vi "cs-scanning_v5_ssx.vi"() -> ()   [LabVIEW 2017]
uses:
  fpga_subVIs_ssxy/fixed-point-ss/typeDefs/FXPControlParams-ss-xy.ctl
  controls/supervisor-params.ctl
  controls/fpga-scan-status.ctl
  controls/boolean_info.ctl
  controls/z-axis-params_v4_prescan.ctl
  controls/TF-params.ctl
  <vilib>/Platform/TimedLoop/XDataNode/timing_clust.ctl
  <vilib>/Platform/TimedLoop/XDataNode/nitl_modes.ctl
  <vilib>/Platform/TimedLoop/XDataNode/wakeup.ctl
  <vilib>/rvi/Emulation/niFpgaGetClockAttributes.vi
  <vilib>/rvi/Emulation/niFpgaSctlEmulationGetInTimedLoop.vi
  <vilib>/rvi/Emulation/niFpgaEmulationReportErrorSimple.vi
  <vilib>/rvi/eio/common/nirviEmuTemplateMethod_errors.vi
  <vilib>/rvi/Emulation/niFpgaCriticalErrorInLSC.vi
  <vilib>/rvi/Memory/Memory_Emulation/nirvimemoryFastEmulation.vi
  <vilib>/rvi/Memory/Memory_Emulation/nirvimemoryEmulation.vi
  <vilib>/rvi/Emulation/niFpgaEmulationIsFPGAContextNoSignature.vi
  <vilib>/rvi/DataTransferAndStorage/Container/Common/niFpgaContainerGetUniqueNameForEmu.vi
  <vilib>/rvi/Emulation/niFpgaProcessEmulError.vi
  <vilib>/rvi/errors/nirviReportUnexpectedCaseInternalError (U32).vi
  <vilib>/rvi/Memory/Memory_Emulation/niFpgaMemoryEmulationCacheClearOnFirstRun.vi
  <vilib>/rvi/Memory/Memory_Emulation/nirvimemoryEmulationManagerCache_MakeExclusive.vi
  <vilib>/rvi/Memory/Memory_Emulation/niFpgaMemoryEmulationValidateCache.vi
  <vilib>/rvi/Memory/Memory_Emulation/nirvimemoryEmulationManagerCache_InsertValue.vi
  <vilib>/Utility/error.llb/Clear Errors.vi
  <vilib>/rvi/Memory/Memory_Emulation/nirvimemoryEmulationManagerCache_ReleaseExclusive.vi
  <vilib>/rvi/Memory/Memory_Emulation/nirvimemoryEmulationManagerCache_GetValue.vi
  <vilib>/rvi/Memory/Memory_Emulation/nirvimemoryEmulationManagerCache_SetValue.vi
  <vilib>/rvi/DataTransferAndStorage/Container/Common/niFpgaContainerExecOnDevCompGetState.vi
  <vilib>/rvi/errors/niFpgaSetErrorForExecOnDevCompSimple.vi
  <vilib>/rvi/eio/common/nirviEmuReportErrorAndStop.vi
  <vilib>/rvi/FIFO/Fifo_Resource/nirvififoEmulationSetSize.vi
  <vilib>/rvi/FIFO/Fifo_Resource/nirviFifoEmulationQueueMgr.vi
  <instcachedir>/0/nirviFifoEmulationQueueMgr_E5CAEC123FF24DC58D834DCA3CDAA9B5.lvgen/nirviFifoEmulationQueueMgr_E5CAEC123FF24DC58D834DCA3CDAA9B5_001.vi
  <vilib>/rvi/FIFO/Fifo_Resource/nirvififoEmulationDetermineInputValidOut.vi
  <vilib>/rvi/FIFO/Fifo_Resource/nirvififoEmulationCreateLock.vi
  <vilib>/rvi/FIFO/Fifo_Resource/nirvififoEmulationObtainLock.vi
  <vilib>/rvi/FIFO/Fifo_Resource/nirvififoEmulationReleaseLock.vi
  <vilib>/rvi/occurrence/nirviWaitOnOccurrenceBase.vi
  <vilib>/rvi/errors/nirviReportUnexpectedCaseInternalError.vi
  <vilib>/rvi/interface/RandomDataEmulation/niFpgaRandomDataHandleErrors.vi
  <vilib>/eio/EIONode/EIONode.xnode
  <vilib>/Platform/TimedLoop/XDataNode/XDataNode.xnode
  <vilib>/rvi/DataTransferAndStorage/Container/XNode/niFpgaContainer.xnode
  <vilib>/rvi/DataTransferAndStorage/Register/Emulation/niFpgaRegisterEmulation.vi
  <vilib>/rvi/FIFO/Fifo_Resource/niFpgaFifoEmulationRefIn.vi
  FPGA-data-logging.lvlib
  libimaging-cs.lvlib
  <vilib>/Platform/TimedLoop/XDataNode/XDNodeRunTimeDep.lvlib
panel:
  in  "collect-0":bool
  out "setup-finished":bool
  out "state0-count":u64
  in  "stop":bool
  out "u_z saturated":bool
  in  "z_axis_params":T1={"z_u_max"=5.0, "setpoint_scan"=0.0, "Ki_scan"=0.001, "uz_safe"=0.0, "Kiz_down"=0.001, "setpoint_up"=0.0, "do_Dz"=FALSE, "PID_while_xy_move"=FALSE, "TF_params"={"TF_order"=0, "Num"=[0.0, 0.0, 0.0, 0.0, 0.0, 0.0, 0.0, 0.0, 0.0], "Den"=[0.0, 0.0, 0.0, 0.0, 0.0, 0.0, 0.0, 0.0, 0.0]}} {"Kiz_down" format="%#_13g"; "z_u_max" format="%#_13g"}
  out "scan-status":T3
  in  "state-machine-params":T5={"xy_settled_samples_threshold"=15, "xy_error_threshold"=0.01, "zup_err_threshold"=0.10000228881835938, "prescan_samples"=5000, "TOL"=0.3, "collect_all"=TRUE, "numEntities"=0} {"TOL" format="%#_13g"}
  in  "num-log-channels":i32
  out "SS FIFO TimeOut?":bool
  in  "ControlParams-ss-xy":T6={"umax"=3.0, "Ns_obs/cntrl"=0, "ref_f_VEC"=[0.0, 0.0], "du_max"=0.0, "Nbar"=0.0, "Nhyst"=0, "Nsat"=0, "Ndrift+1"=0, "Ki-y"=0.01}
  out "loop-stopped":bool
  out "xyZ_k":fxp<+/-,16,5>[](array[numeric])
  out "xy_ref":fxp<+/-,16,5>[](array[numeric])
  out "u_x saturated":bool
  out "u_y saturated":bool
  out "scan-idx":i16
  out "number-settled-samples-Z":i16
  out "current-state":u8
  out "z-u(k)":fxp<+/-,16,5>
  in  "ABORT":bool
  out "read fifo timeout":bool
  in  "trigger-0":bool
  out "number-settled-samples-y":i16
  out "number-settled-samples-x":i16
  # "- If collect all = fasle ,\nwe only collect measurement data.\n- If collect all = true, we collect everything."
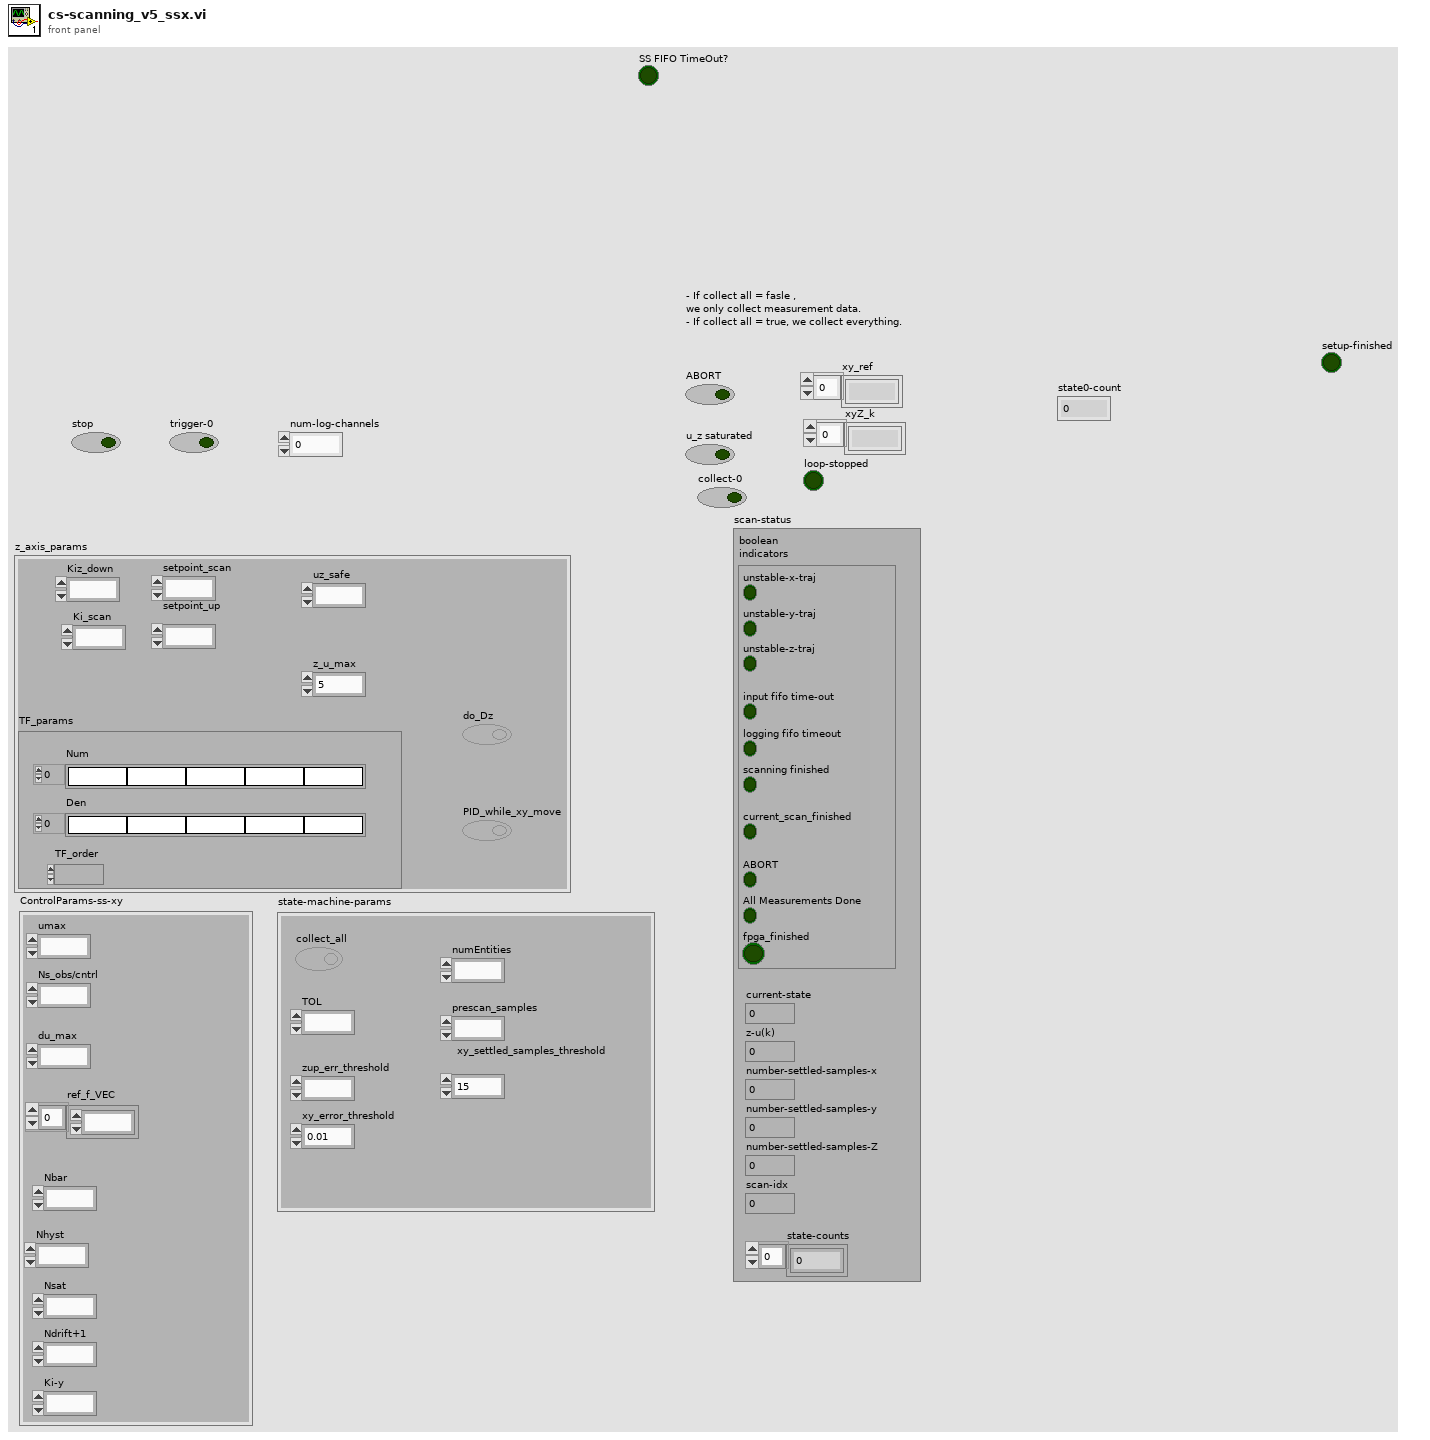
[diagram p1: front panel]
types:
  T1 = typedef "z-axis-params_v4_prescan.ctl" = cluster{"z_u_max":sgl, "setpoint_scan":fxp<+/-,32,16>, "Ki_scan":sgl, "uz_safe":fxp<+/-,16,5>, "Kiz_down":sgl, "setpoint_up":fxp<+/-,32,16>, "do_Dz":bool, "PID_while_xy_move":bool, "TF_params":T2}
  T2 = typedef "TF-params.ctl" = cluster{"TF_order":i16, "Num":sgl[], "Den":sgl[]}
  T3 = typedef "fpga-scan-status.ctl" = cluster{"boolean \nindicators":T4, "current-state":u8, "z-u(k)":sgl, "number-settled-samples-x":i16, "number-settled-samples-y":i16, "number-settled-samples-Z":i16, "scan-idx":i16, "state-counts":u64[]}
  T4 = typedef "boolean_info.ctl" = cluster{"unstable-z-traj":bool, "input fifo time-out":bool, "logging fifo timeout":bool, "scanning finished":bool, "unstable-x-traj":bool, "unstable-y-traj":bool, "ABORT":bool, "All Measurements Done":bool, "fpga_finished":bool, "current_scan_finished":bool}
  T5 = typedef "supervisor-params.ctl" = cluster{"xy_settled_samples_threshold":i16, "xy_error_threshold":sgl, "zup_err_threshold":fxp<+,24,5>, "prescan_samples":i16, "TOL":sgl, "collect_all":bool, "numEntities":i16}
  T6 = typedef "FXPControlParams-ss-xy.ctl" = cluster{"umax":fxp<+/-,18,5>, "Ns_obs/cntrl":u8, "ref_f_VEC":fxp<+/-,32,5>[], "du_max":fxp<+/-,18,5>, "Nbar":fxp<+/-,32,5>, "Nhyst":u8, "Nsat":u8, "Ndrift+1":u8, "Ki-y":sgl}
  T7 = typedef "XDNodeRunTimeDep.lvlib/timing_clust.ctl" = cluster{"Expected End [f-1]":u64, "Actual End [f-1]":u64, "Finished Late? [f-1]":bool, "Expected End [i-1]":u64, "Actual End [i-1]":u64, "Finished Late? [i-1]":bool, "Expected Start [i]":u64, "Actual Start [i]":u64, "Expected Start [f]":u64, "Actual Start [f]":u64, "Source Name":string, "Structure Name":string, "Period":i64, "Deadline":i64, "Offset":i64, "Start":i64, "Priority":i32, "Timeout":i32, "Mode":T8, "Wakeup Reason":T9, "Error":errorcluster, "Source Type":string, "Secondary Source Type":string, "Global End Time":u64, "Global Start Time":u64, "Frame Duration":u64, "Iteration Duration":u64, "Assigned CPU":i32, "I/O Scan Engine Mode":u32}
  T8 = typedef "XDNodeRunTimeDep.lvlib/nitl_modes.ctl" = enum32{"No Change", "Process missed periods, maintain original phase", "Discard missed periods, maintain original phase", "Process missed periods, ignore original phase", "Discard missed periods, ignore original phase"}
  T9 = typedef "XDNodeRunTimeDep.lvlib/wakeup.ctl" = enum32{"Normal", "Aborted", "Asynchronous wakeup", "Timing source error", "Timed loop error", "Timeout"}
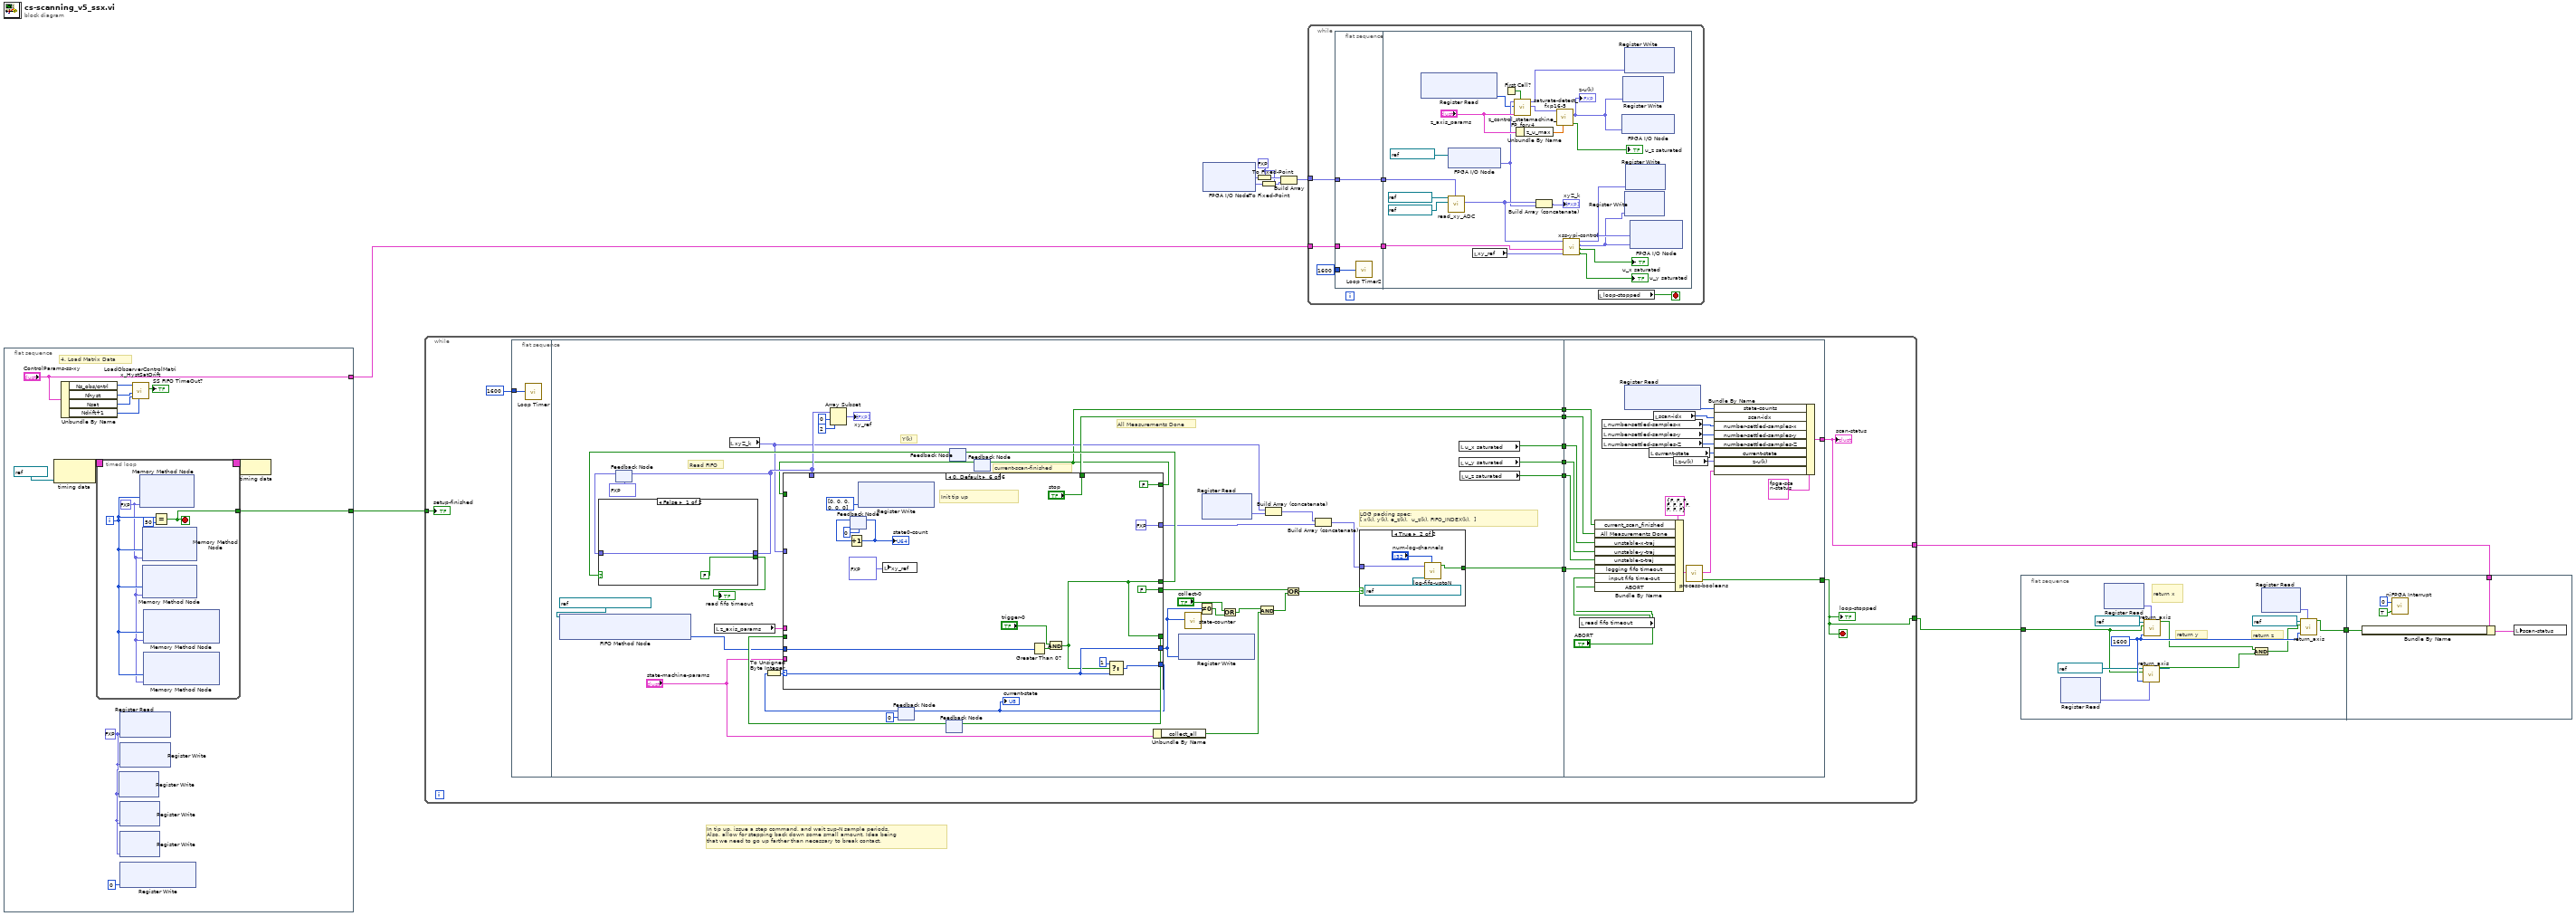
[diagram p0: block diagram]
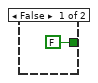
[diagram p2: hidden frame]
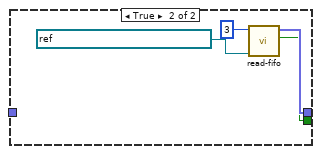
[diagram p3: hidden frame]
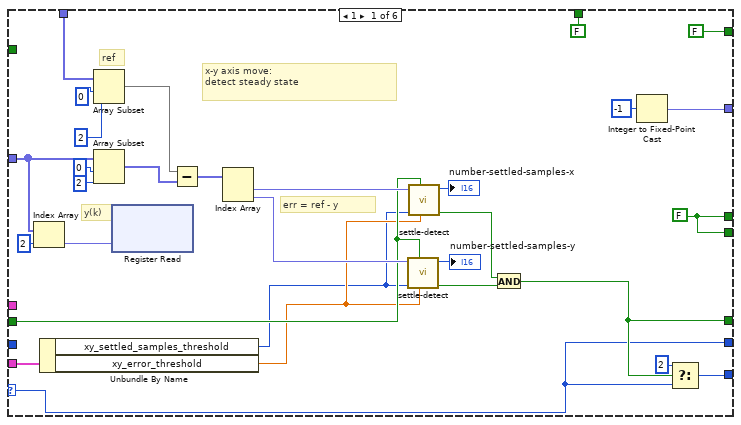
[diagram p4: hidden frame]
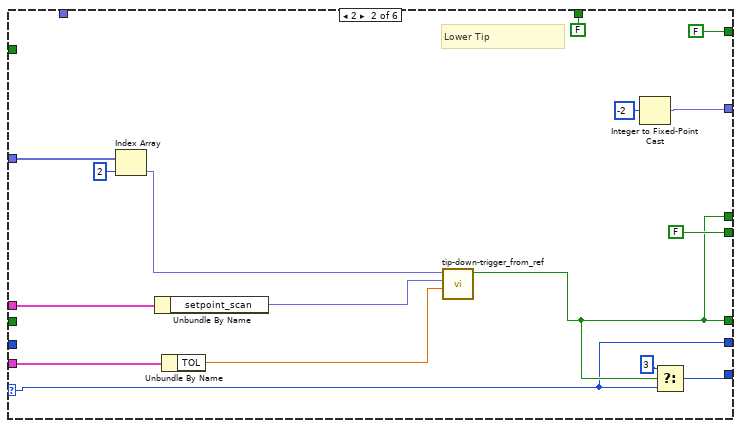
[diagram p5: hidden frame]
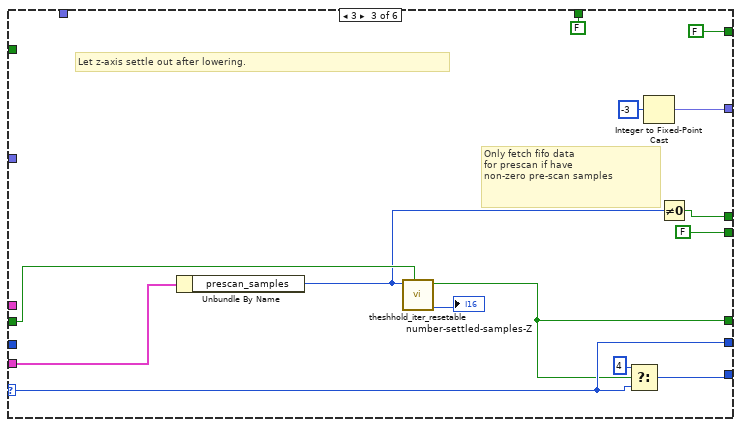
[diagram p6: hidden frame]
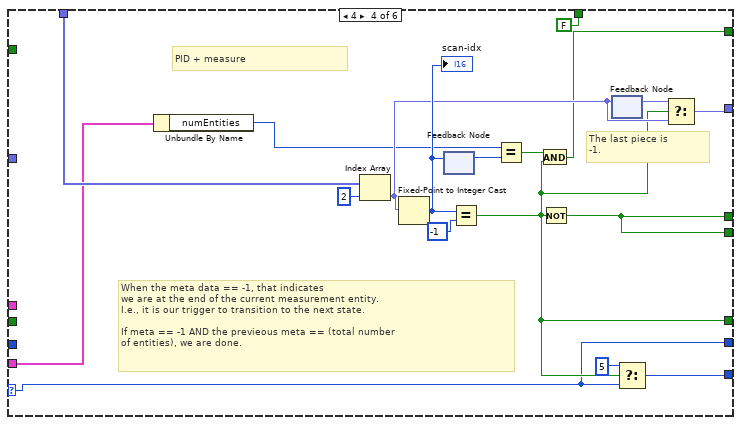
[diagram p7: hidden frame]
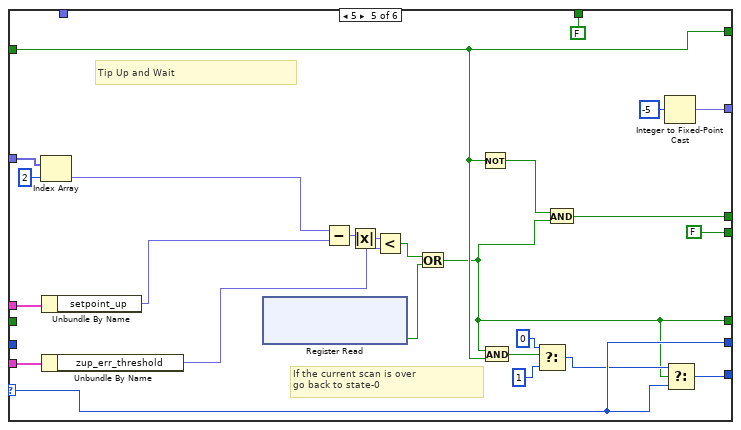
[diagram p8: hidden frame]
diagram:
  w5 = fxp<+/-,16,5> 0.0 ("fixed-point type")
  # "In tip up, issue a step command, and wait zup-N sample periods.\nAlso, allow for stepping back down some small amount. Idea being \nthat we need to go up farther than necessary to break contact."
  n1 = flat-sequence {
    tunnel: ["ControlParams-ss-xy"] -> w4
    tunnel: [w12] -> w1
    frame #0 {
      w14 = fxp<+/-,16,5> 0.0 ("Data")
      # "4. Load Matrix Data"
      n2 = node-c288(refnum<k21> "80MHz" ("Source Name")) -> (w23:T7)
      n3 = Unbundle By Name("ControlParams-ss-xy") -> ("Ns_obs/cntrl"=w20:u8, "Nhyst"=w18:u8, "Nsat"=w17:u8, "Ndrift+1"=w16:u8)
      n4 = timed-loop {
        timing: w23 -> [_]
        timing-out: [_] -> w22
        tunnel: [w24] -> w12
        i -> [w26]
        stop <- w24 stop-if-true
        w25 = fxp<+/-,32,5> 0.0 ("Data")
        n5 = xnode ("Memory Method Node")("Address"=w26, "Data"=w25) -> ()  [unwired: 1 in, 1 out]
        n6 = xnode ("Memory Method Node")("Address"=w26, "Data"=w25) -> ()  [unwired: 1 in, 1 out]
        n7 = xnode ("Memory Method Node")("Address"=w26, "Data"=w25) -> ()  [unwired: 1 in, 1 out]
        n8 = xnode ("Memory Method Node")("Address"=w26, "Data"=w25) -> ()  [unwired: 1 in, 1 out]
        n9 = xnode ("Memory Method Node")("Address"=w26, "Data"=w25) -> ()  [unwired: 1 in, 1 out]
        n10 = Equal?(x=w26, y=50) -> (x = y?=w24:bool)
      }
      n11 = xnode ("Register Write")("Data"=w14) -> ()  [unwired: 1 in, 1 out]
      n12 = xnode ("Register Write")("Data"=w14) -> ()  [unwired: 1 in, 1 out]
      n13 = xnode ("Register Write")("Data"=w14) -> ()  [unwired: 1 in, 1 out]
      n14 = xnode ("Register Write")("Data"=u8 0) -> ()  [unwired: 1 in, 1 out]
      n15 = xnode ("Register Read")("Data"=w14) -> ()  [unwired: 1 in, 1 out]
      n16 = xnode ("Register Write")("Data"=w14) -> ()  [unwired: 1 in, 1 out]
      n17 = call "LoadObserverControlMatrix_HystSatDrift.vi"("Ndrift+1"=w16, "Nsat"=w17, "Nhyst"=w18, "NS_obs/cntrl"=w20) -> ("SS FIFO TimeOut?"=→"SS FIFO TimeOut?":bool)  [unwired: 7 in]
      n18 = node-c288(w22) -> ()
    }
  }
  n19 = while {
    tunnel: [w39] -> w11
    tunnel: [w37] -> w2
    tunnel: w1 -> [w35]
    stop <- w37 stop-if-true
    n20 = flat-sequence {
      tunnel: u32 1600 ("TsTicks") -> [w44]
      tunnel: [w81] -> w43
      tunnel: [w71] -> w42
      tunnel: [w68] -> w41
      tunnel: [w67] -> w40
      tunnel: [w57] -> w36
      tunnel: [w47] -> w34
      tunnel: w43 -> [w232]
      tunnel: w42 -> [w229]
      tunnel: [w228] -> w37
      tunnel: w41 -> [w227]
      tunnel: w40 -> [w226]
      tunnel: [w217] -> w39
      tunnel: w36 -> [w216]
      tunnel: w34 -> [w214]
      frame #0 {
        n21 = call "Loop Timer"("Count(Ticks)"=w44) -> ()  [unwired: 1 out]
      }
      frame #1 {
        # "current-scan-finished"
        # "All Measurements Done"
        # "Y(k)"
        # "LOG packing spec:\n[ x(k), y(k), e_z(k),  u_z(k), FIFO_INDEX(k),  ]"
        # "Read FIFO"
        n22 = xnode ("FIFO Method Node")("FIFO In"=refnum<k21> "host-to-fpga-fxp-16-5") -> ("Number of Elements to Read"=w45:u32)  [unwired: 1 out]
        n23 = feedback #1(fxp<+/-,16,5>[] [0.0, 0.0, 0.0] ("unpacked-data")) -> (w83:fxp<+/-,16,5>[])
        n24 = local read "z_axis_params"() -> (w55:T1)
        n25 = local read "xyZ_k"() -> (w54:fxp<+/-,16,5>[])
        n26 = feedback #2(u8 0 ("t")) -> (w62:u8)
        n27 = To Unsigned Byte Integer(number=w62) -> (unsigned 8bit integer=w63:u8)
        n28 = feedback #3() -> (w75:bool)  [unwired: 1 in]
        n29 = feedback #4() -> (w78:bool)  [unwired: 1 in]
        n30 = case shown="False" w78 {
          tunnel: w83 -> [w90 _]
          tunnel: [w90 w93] -> w59
          tunnel: [FALSE ("timout?") w92] -> w80
          frame False {
          }
          frame True {
            n31 = call "read-fifo.vi"("FIFO In"=refnum<k21> "host-to-fpga-fxp-16-5", "numChan"=3) -> ("timout?"=w92:bool, "unpacked-data"=w93:fxp<+/-,16,5>[])  [unwired: 8 in]
          }
        }
        "read fifo timeout" <- w80
        n32 = feedback-in #1(w59) -> ()
        n33 = Array Subset(array=w59, index=0, length=2) -> (→"xy_ref":fxp<+/-,16,5>[])
        n34 = feedback #5() -> (w52:bool)  [unwired: 1 in]
        n35 = case shown="0, Default" w63 {
          selector: w63 -> [w99 w129 w147 w158 w191 w208]
          tunnel: [w100 FALSE FALSE ("trigger-0") w164 FALSE FALSE] -> w72
          tunnel: [w119 w137 w153 w171 w196 w213] -> w61
          tunnel: w54 -> [w101 w139 _ _ w192 _]
          tunnel: [w100 w130 w142 w164 w178 w200] -> w79
          tunnel: [FALSE FALSE FALSE FALSE FALSE "stop"] -> w71
          tunnel: w59 -> [w110 _ _ w166 _ _]
          tunnel: w75 -> [w108 _ w148 _ _ _]
          tunnel: [w107 w130 w146 w160 w173 w200] -> w76
          tunnel: [w104 w131 w149 w163 w194 fxp<+/-,16,5> 0.0 ("Element")] -> w64
          tunnel: [w99 w129 w147 w158 w191 w208] -> w53
          tunnel: "state-machine-params" -> [w98 w128 w144 w157 w186 _]
          tunnel: w55 -> [_ w126 _ _ w184 _]
          tunnel: w52 -> [_ _ _ _ w176 _]
          tunnel: [FALSE FALSE FALSE w155 w176 FALSE] -> w47
          tunnel: w45 -> [_ _ _ _ _ w198]
          frame 1 {
            w100 = FALSE
            # "y(k)"
            # "err = ref - y"
            # "ref"
            # "x-y axis move: \ndetect steady state"
            n36 = Index Array(array=w101, index=2) -> (element=w103:fxp<+/-,16,5>)
            n37 = Unbundle By Name(w98) -> ("xy_settled_samples_threshold"=w96:i16, "xy_error_threshold"=w97:sgl)
            n38 = Array Subset(array=w110, index=0, length=2) -> (w114:fxp<+/-,16,5>[])
            n39 = Array Subset(array=w101, index=0, length=2) -> (w113:fxp<+/-,16,5>[])
            n40 = xnode ("Register Read")("Data"=w103) -> ()  [unwired: 1 in, 1 out]
            n41 = Subtract(x=w114, y=w113) -> (x-y=w106:fxp<+/-,17,6>[])
            n42 = Index Array(array=w106) -> (element #1=w112:fxp<+/-,17,6>, element #2=w111:fxp<+/-,17,6>)  [unwired: 2 in]
            n43 = call "settle-detect.vi"("error-max"=w97, "reset"=w108, "settled-samples\nthreshold"=w96, "err(k)"=w111) -> ("has-settled"=w124:bool, "number-settled-samples"=→"number-settled-samples-y":u16)  [unwired: 6 in]
            n44 = call "settle-detect.vi"("error-max"=w97, "reset"=w108, "settled-samples\nthreshold"=w96, "err(k)"=w112) -> ("has-settled"=w123:bool, "number-settled-samples"=→"number-settled-samples-x":u16)  [unwired: 6 in]
            n45 = And(x=w123, y=w124) -> (x .and. y?=w107:bool)
            n46 = Integer to Fixed-Point Cast(integer=i16 -1) -> (fixed-point=w104:fxp<+/-,16,5>)  [unwired: 1 in]
            n47 = Select(t=u8 2, s=w107, f=w99) -> (s? t:f=w119:u8)
          }
          frame 2 {
            # "Lower Tip"
            n48 = Index Array(array=w139, index=2) -> (element=w138:fxp<+/-,16,5>)
            n49 = Unbundle By Name(w126) -> ("setpoint_scan"=w132:fxp<+/-,32,16>)
            n50 = Unbundle By Name(w128) -> ("TOL"=w127:sgl)
            n51 = call "tip-down-trigger_from_ref.vi"("TOL"=w127, "setpoint"=w132, "I/O Item"=w138) -> ("Boolean"=w130:bool)  [unwired: 8 in]
            n52 = Integer to Fixed-Point Cast(integer=i16 -2) -> (fixed-point=w131:fxp<+/-,16,5>)  [unwired: 1 in]
            n53 = Select(t=u8 3, s=w130, f=w129) -> (s? t:f=w137:u8)
          }
          frame 3 {
            # "Only fetch fifo data\nfor prescan if have\nnon-zero pre-scan samples"
            # "Let z-axis settle out after lowering."
            n54 = Unbundle By Name(w144) -> ("prescan_samples"=w141:i16)
            n55 = call "theshhold_iter_resetable.vi"("reset"=w148, "N"=w141) -> ("iter"=→"number-settled-samples-Z":i16, "Boolean"=w146:bool)  [unwired: 8 in]
            n56 = Select(t=u8 4, s=w146, f=w147) -> (s? t:f=w153:u8)
            n57 = Integer to Fixed-Point Cast(integer=i16 -3) -> (fixed-point=w149:fxp<+/-,16,5>)  [unwired: 1 in]
            n58 = Not Equal To 0?(x=w141) -> (x != 0?=w142:bool)
          }
          frame 4 {
            # "The last piece is\n-1."
            # "When the meta data == -1, that indicates\nwe are at the end of the current measurement entity.\nI.e., it is our trigger to transition to the next state.\n\nIf meta == -1 AND the previeous meta == (total number\nof entities), we are done."
            # "PID + measure"
            n59 = Unbundle By Name(w157) -> ("numEntities"=w156:i16)
            n60 = Index Array(array=w166, index=2) -> (element=w161:fxp<+/-,16,5>)
            n61 = Fixed-Point to Integer Cast(1:w161) -> (0:w165:i16)
            "scan-idx" <- w165
            n62 = feedback #6() -> (w167:i16)  [unwired: 1 in]
            n63 = feedback-in #6(w165) -> ()
            n64 = Equal?(x=w165, y=i16 -1) -> (x = y?=w160:bool)
            n65 = Equal?(x=w156, y=w167) -> (x = y?=w168:bool)
            n66 = And(x=w168, y=w160) -> (x .and. y?=w155:bool)
            n67 = Not(x=w160) -> (.not. x?=w164:bool)
            n68 = feedback #7() -> (w162:fxp<+/-,16,5>)  [unwired: 1 in]
            n69 = feedback-in #7(w161) -> ()
            n70 = Select(t=u8 5, s=w160, f=w158) -> (s? t:f=w171:u8)
            n71 = Select(t=w162, s=w160, f=w161) -> (s? t:f=w163:fxp<+/-,16,5>)
          }
          frame 5 {
            # "If the current scan is over\ngo back to state-0"
            # "Tip Up and Wait"
            n72 = Index Array(array=w192, index=2) -> (element=w190:fxp<+/-,16,5>)
            n73 = Unbundle By Name(w184) -> ("setpoint_up"=w187:fxp<+/-,32,16>)
            n74 = Unbundle By Name(w186) -> ("zup_err_threshold"=w185:fxp<+,24,5>)
            n75 = xnode ("Register Read")() -> ("Data"=w174:bool)  [unwired: 1 in, 1 out]
            n76 = Subtract(x=w190, y=w187) -> (x-y=w189:fxp<+/-,33,17>)
            n77 = Absolute Value(x=w189) -> (abs(x)=w188:fxp<+,32,16>)
            n78 = Less?(x=w188, y=w185) -> (x < y?=w175:bool)
            n79 = Or(x=w175, y=w174) -> (x .or. y?=w173:bool)
            n80 = Not(x=w176) -> (.not. x?=w177:bool)
            n81 = And(x=w173, y=w176) -> (x .and. y?=w182:bool)
            n82 = Select(t=u8 0, s=w182, f=u8 1) -> (s? t:f=w179:u8)
            n83 = And(x=w177, y=w173) -> (x .and. y?=w178:bool)
            n84 = Integer to Fixed-Point Cast(integer=i16 -5) -> (fixed-point=w194:fxp<+/-,16,5>)  [unwired: 1 in]
            n85 = Select(t=w179, s=w173, f=w191) -> (s? t:f=w196:u8)
          }
          frame 0, Default {
            # "Init tip up"
            n86 = feedback #8(u64 0) -> (w205:u64)
            n87 = Increment(x=w205) -> (x+1=w206:u64)
            "state0-count" <- w206
            n88 = feedback-in #8(w206) -> ()
            n89 = xnode ("Register Write")("Data"=u64[] [0, 0, 0, 0, 0, 0]) -> ()  [unwired: 1 in, 1 out]
            n90 = local write "xy_ref"(fxp<+/-,16,5>[] [0.0, 0.0] ("xy_ref")) -> ()
            n91 = Greater Than 0?(x=w198) -> (x > 0?=w199:bool)
            n92 = And(x="trigger-0", y=w199) -> (x .and. y?=w200:bool)
            n93 = Select(t=u8 1, s=w200, f=w208) -> (s? t:f=w213:u8)
          }
        }
        "current-state" <- w61
        n94 = feedback-in #2(w61) -> ()
        n95 = feedback-in #3(w76) -> ()
        n96 = feedback-in #4(w79) -> ()
        n97 = feedback-in #5(w47) -> ()
        n98 = Unbundle By Name("state-machine-params") -> ("collect_all"=w58:bool)
        n99 = xnode ("Register Write")("Data"=w53) -> ()  [unwired: 1 in, 1 out]
        n100 = call "state-counter.vi"("state-idx"=w53) -> ()  [unwired: 11 in]
        n101 = Not Equal To 0?(x=w53) -> (x != 0?=w49:bool)
        n102 = xnode ("Register Read")() -> ("Data"=w56:fxp<+/-,16,5>)  [unwired: 1 in, 1 out]
        n103 = Or(x="collect-0", y=w49) -> (x .or. y?=w50:bool)
        n104 = And(x=w50, y=w58) -> (x .and. y?=w73:bool)
        n105 = Build Array (concatenate)(w54, w56) -> (w65:fxp<+/-,16,5>[])
        n106 = Or(x=w72, y=w73) -> (x .or. y?=w74:bool)
        n107 = Build Array (concatenate)(w65, w64) -> (w82:fxp<+/-,16,5>[])
        n108 = case shown="True" w74 {
          tunnel: w82 -> [_ w88]
          tunnel: [FALSE ("logging-timeout?") w87] -> w81
          frame False {
          }
          frame True {
            n109 = call "log-fifo-uptoN.vi"("N"="num-log-channels", "FIFO In"=refnum<k21> "fpga-to-host2-fxp-16-5", "input-data"=w88) -> ("logging-timeout?"=w87:bool)  [unwired: 8 in]
          }
        }
        n110 = local read "u_x saturated"() -> (w68:bool)
        n111 = local read "u_y saturated"() -> (w67:bool)
        n112 = local read "u_z saturated"() -> (w57:bool)
      }
      frame #2 {
        n113 = local read "read fifo timeout"() -> (w231:bool)
        n114 = Bundle By Name(cluster=T4 {"unstable-z-traj"=FALSE, "input fifo time-out"=FALSE, "logging fifo timeout"=FALSE, "scanning finished"=FALSE, "unstable-x-traj"=FALSE, "unstable-y-traj"=FALSE, "ABORT"=FALSE, "All Measurements Done"=FALSE, "fpga_finished"=FALSE, "current_scan_finished"=FALSE} ("boolean errors"), "current_scan_finished"=w214, "All Measurements Done"=w229, "unstable-x-traj"=w227, "unstable-y-traj"=w226, "unstable-z-traj"=w216, "logging fifo timeout"=w232, "input fifo time-out"=w231, "ABORT"="ABORT") -> (w233:T4)
        n115 = local read "number-settled-samples-x"() -> (w220:i16)
        n116 = local read "number-settled-samples-y"() -> (w221:i16)
        n117 = local read "number-settled-samples-Z"() -> (w222:i16)
        n118 = xnode ("Register Read")() -> ("Data"=w215:u64[])  [unwired: 1 in, 1 out]
        n119 = local read "current-state"() -> (w224:u8)
        n120 = local read "scan-idx"() -> (w219:i16)
        n121 = local read "z-u(k)"() -> (w225:fxp<+/-,16,5>)
        n122 = call "process-booleans.vi"("boolean indicators 2"=w233) -> ("scaning finished"=w228:bool, "boolean indicators"=w223:T4)  [unwired: 9 in]
        n123 = Bundle By Name(cluster=T3 {"boolean \nindicators"={"unstable-z-traj"=FALSE, "input fifo time-out"=FALSE, "logging fifo timeout"=FALSE, "scanning finished"=FALSE, "unstable-x-traj"=FALSE, "unstable-y-traj"=FALSE, "ABORT"=FALSE, "All Measurements Done"=FALSE, "fpga_finished"=FALSE, "current_scan_finished"=FALSE}, "current-state"=0, "z-u(k)"=0.0, "number-settled-samples-x"=0, "number-settled-samples-y"=0, "number-settled-samples-Z"=0, "scan-idx"=0, "state-counts"=[0, 0, 0, 0, 0, 0]} ("input cluster"), "state-counts"=w215, "scan-idx"=w219, "number-settled-samples-x"=w220, "number-settled-samples-y"=w221, "number-settled-samples-Z"=w222, "current-state"=w224, "z-u(k)"=w225, "boolean \nindicators"=w223) -> (w217:T3)
      }
    }
    "loop-stopped" <- w37
    "scan-status" <- w39
    "setup-finished" <- w35
  }
  n124 = xnode "FPGA I/O Node"() -> ("Mod2/AI0"=w9:fxp<+/-,24,5>, "Mod2/AI1"=w7:fxp<+/-,24,5>)  [unwired: 2 in, 2 out]
  n125 = To Fixed-Point(fixed-point type=w5, number=w9) -> (fixed-point=w10:fxp<+/-,16,5>)
  n126 = To Fixed-Point(fixed-point type=w5, number=w7) -> (fixed-point=w8:fxp<+/-,16,5>)
  n127 = Build Array(w10, w8) -> (w6:fxp<+/-,16,5>[])
  n128 = while {
    tunnel: w6 -> [w235]
    tunnel: w4 -> [w238]
    stop <- w240 stop-if-true
    n129 = flat-sequence {
      tunnel: u32 1600 ("TsTicks") -> [w243]
      tunnel: [w242] -> w239
      tunnel: w238 -> [w242]
      tunnel: [w241] -> w236
      tunnel: w235 -> [w241]
      tunnel: w239 -> [w259]
      tunnel: w236 -> [w256]
      frame #0 {
        n130 = call "Loop Timer2"("Count(Ticks)"=w243) -> ()  [unwired: 1 out]
      }
      frame #1 {
        n131 = xnode ("Register Read")() -> ("Data"=w249:u8)  [unwired: 1 in, 1 out]
        n132 = xnode "FPGA I/O Node"("FPGA I/O In"=refnum<k21> "Mod2/AI2" ("y - ADC")) -> ("I/O Item"=w251:fxp<+/-,24,5>)  [unwired: 1 out]
        n133 = call "read_xy_ADC.vi"("x(0), y(0)"=w256, "y - ADC"=refnum<k21> "Mod2/AI1", "x - ADC"=refnum<k21> "Mod2/AI0") -> ("x_y"=w252:fxp<+/-,17,6>[])  [unwired: 8 in]
        n134 = local read "xy_ref"() -> (w262:fxp<+/-,16,5>[])
        n135 = First Call?() -> (First Call?: T/F=w248:bool)
        n136 = call "z_control_statemachine_FP_forv4.vi"("reset-PI"=w248, "z_axis_params"="z_axis_params", "State"=w249, "zerr(k)"=w251) -> ("zuk_Dinv"=w247:fxp<+/-,16,5>, "z-u(k)"=w254:fxp<+/-,16,5>)  [unwired: 6 in]
        n137 = Unbundle By Name("z_axis_params") -> ("z_u_max"=w245:sgl)
        n138 = Build Array (concatenate)(w252, w251) -> (→"xyZ_k":fxp<+/-,25,6>[])
        n139 = call "saturate-detect_fxp16-5.vi"("bound"=w245, "x"=w247) -> ("saturated"=→"u_z saturated":bool, "sat(x)"=w244:fxp<+/-,16,5>)  [unwired: 8 in]
        "z-u(k)" <- w244
        n140 = call "xss-ypi-control.vi"("xy-ref"=w262, "ControlParamsLin"=w259, "x_k-y_k"=w252) -> ("u_y saturated"=→"u_y saturated":bool, "u_x saturated"=→"u_x saturated":bool, "sat(u_y)"=w257:fxp<+/-,18,5>, "u_k (saturated)"=w258:fxp<+/-,32,5>)  [unwired: 5 in]
        n141 = xnode "FPGA I/O Node"("Mod1/AO2"=w244) -> ()  [unwired: 1 in, 1 out]
        n142 = xnode ("Register Write")("Data"=w244) -> ()  [unwired: 1 in, 1 out]
        n143 = xnode ("Register Write")("Data"=w254) -> ()  [unwired: 1 in, 1 out]
        n144 = xnode ("Register Write")("Data"=w257) -> ()  [unwired: 1 in, 1 out]
        n145 = xnode ("Register Write")("Data"=w258) -> ()  [unwired: 1 in, 1 out]
        n146 = xnode "FPGA I/O Node"("Mod1/AO0"=w258, "Mod1/AO1"=w257) -> ()  [unwired: 2 in, 2 out]
      }
    }
    n147 = local read "loop-stopped"() -> (w240:bool)
  }
  n148 = flat-sequence {
    tunnel: [w268] -> w3
    tunnel: w2 -> [w267]
    tunnel: w11 -> [w281]
    tunnel: w3 -> [w280]
    frame #0 {
      w276 = i16 1600
      # "return z"
      # "return y"
      # "return x"
      n149 = xnode ("Register Read")() -> ("Data"=w272:fxp<+/-,16,5>)  [unwired: 1 in, 1 out]
      n150 = xnode ("Register Read")() -> ("Data"=w271:fxp<+/-,16,5>)  [unwired: 1 in, 1 out]
      n151 = call "return_axis.vi"("u(0)"=w272, "TsTicks"=w276, "phony-enable"=w267, "FPGA I/O In"=refnum<k21> "Mod1/AO1") -> ("finished"=w265:bool)  [unwired: 7 in]
      n152 = call "return_axis.vi"("u(0)"=w271, "TsTicks"=w276, "phony-enable"=w267, "FPGA I/O In"=refnum<k21> "Mod1/AO0") -> ("finished"=w266:bool)  [unwired: 7 in]
      n153 = And(x=w266, y=w265) -> (x .and. y?=w270:bool)
      n154 = xnode ("Register Read")() -> ("Data"=w269:fxp<+/-,16,5>)  [unwired: 1 in, 1 out]
      n155 = call "return_axis.vi"("u(0)"=w269, "TsTicks"=w276, "phony-enable"=w270, "FPGA I/O In"=refnum<k21> "Mod1/AO2") -> ("finished"=w268:bool)  [unwired: 7 in]
    }
    frame #1 {
      n156 = Bundle By Name(cluster=w281, "boolean \nindicators.fpga_finished"=w280) -> (w279:T3)
      n157 = call <vilib>:"niFPGA Interrupt.vi"("Wait Until Cleared (F)"=TRUE, "IRQ Number (0)"=u8 0) -> ()  [unwired: 1 in]
      n158 = local write "scan-status"(w279) -> ()
    }
  }
